vi "GUI_MicrophoneTest.vi"() -> ()   [LabVIEW 2018]
uses:
  C:/Micriphone Test/Microfontest/Peiker_Stepped Sweep Settings.ctl
  <vilib>/addons/_NISVFA/_Shared subVIs/Controls/svc_DSA Channel Settings.ctl
  <vilib>/addons/_NISVFA/_Shared subVIs/Controls/svc_Channel Info.ctl
  <vilib>/addons/_NISVFA/_Shared subVIs/Controls/svc_Engineering Units Text Ring.ctl
  <vilib>/addons/_NISVFA/_Shared subVIs/Controls/svc_Weighting Filter Text Ring.ctl
  <vilib>/addons/Sound and Vibration/svt_Limit Test/SVL Limit Testing (XY) (scalar limits).vi
  <vilib>/addons/Sound and Vibration/svt_Limit Test/SoundVib_LimitTest.lvlib
panel:
  in  "Input Settings.Responce Channel Settings.response channel info":T1={"sensor sensitivity"=1000.0, "engineering units"=1, "dB reference"=1.0, "custom label"="EU", "weighting filter"=0, "pregain"=0.0} {"pregain" format="%.2f"; "weighting filter" items=["Linear", "A-weighting", "B-weighting", "C-weighting", "ITU-R 468-4", "Dolby", "CCITT", "C-message", "Wb", "Wc", "Wd", "We", "Wf", "Wh", "Wj", "Wk", "Wm", "AES17 20 kHz lowpass", "AES17 40 kHz lowpass", "AES17 20 kHz highpass", "AES17 40 kHz highpass"]; "dB reference" format="%^.1e"; "engineering units" items=["custom..."=0, "V"=1, "A"=21, "C"=30, "pC"=31, "s"=32, "-"=29, "Pa"=2, "N"=20, "g"=3, "m/s^2"=4, "m/s"=5, "m"=6, "mm/s"=12, "mm"=13, "micron/s"=14, "micron"=15, "in/s^2"=7, "in/s"=8, "in"=9, "mil/s"=10, "mil"=11, "rad/s^2"=16, "rad/s"=17, "rad"=18, "deg/s^2"=26, "deg/s"=27, "deg"=28, "RPM"=22, "cycle/s^2"=23, "Hz"=24, "cycle"=25, "strain"=19]; "sensor sensitivity" format="%#_5f"}
  out "Fundamental-Response RMS (Engineering unit) 2":T4(graph)={"frequency [Hz]"=[100.0], "amplitude"=[6.209838309826431]} caption="Fundamental-Response RMS"
  out "THD%":cluster{"frequency":dbl[], "THD":dbl[]} {"THD" format="%.2f"; "frequency" format="%.2f"}
  out "THD-Response":cluster{"frequency":dbl[], "THD":dbl[]}(graph)={"frequency"=[100.0], "THD"=[0.18625048733429]} caption="THD"
  out "Fundamental-Response RMS (Engineering unit)":T4
  in  "THD Frequency":dbl
  out "Fundamental-Response RMS (Engineering unit)":T4(graph) caption="harmonics"
  in  "THD Level (dBSpl)":dbl=94.0
  out "Sensitivity(V)":dbl
  in  "Ref.Frequency":dbl=100.0
  out "magnitude first measurement":dbl[](array[numeric])
  in  "Set level (dBSPL)":i32=94
  in  "Peiker_Stepped Sweep Settings":T5={"Input Settings"={"IEPE min time to settle [s]"=5.0, "Responce Channel Settings"={"DSA response channel settings"={"coupling"=10045, "enable IEPE excitation"=FALSE, "IEPE current [mA]"=4.0}, "response channel info"={"sensor sensitivity"=200.0, "engineering units"=2, "dB reference"=2e-05, "custom label"="EU", "weighting filter"=0, "pregain"=0.0}, "AI response settings"={"response channel"="SOUNDACQ/ai1", "max value [V]"=10.0, "min value [V]"=-10.0, "terminal configuration"=-1}}, "Stimulus Channel Settings"={"AI stimulus settings"={"stimulus channel"="SOUNDACQ/ai0", "max value [V]"=0.15, "min value [V]"=-0.15, "terminal configuration"=-1}, "DSA stimulus channel settings"={"coupling"=10045, "enable IEPE excitation"=TRUE, "IEPE current [mA]"=4.0}, "stimulus channel info"={"sensor sensitivity"=11.4, "engineering units"=2, "dB reference"=2e-05, "custom label"="EU", "weighting filter"=0, "pregain"=0.0}}}, "Output Settings"={"AO source settings"={"excitation channel"="SOUNDACQ/ao0", "max value [V]"=10.0, "min value [V]"=-10.0, "terminal configuration"=-1}}} {"Output Settings"."AO source settings"."terminal configuration" items=["Default"=-1, "RSE"=10083, "Differential"=10106, "Pseudodifferential"=12529]; "Output Settings"."AO source settings"."min value [V]" format="%0.2f"; "Output Settings"."AO source settings"."max value [V]" format="%0.2f"; "Input Settings"."Stimulus Channel Settings"."stimulus channel info"."pregain" format="%.2f"; "Input Settings"."Stimulus Channel Settings"."stimulus channel info"."weighting filter" items=["Linear", "A-weighting", "B-weighting", "C-weighting", "ITU-R 468-4", "Dolby", "CCITT", "C-message", "Wb", "Wc", "Wd", "We", "Wf", "Wh", "Wj", "Wk", "Wm", "AES17 20 kHz lowpass", "AES17 40 kHz lowpass", "AES17 20 kHz highpass", "AES17 40 kHz highpass"]; "Input Settings"."Stimulus Channel Settings"."stimulus channel info"."dB reference" format="%^.1e"; "Input Settings"."Stimulus Channel Settings"."stimulus channel info"."engineering units" items=["custom..."=0, "V"=1, "A"=21, "C"=30, "pC"=31, "s"=32, "-"=29, "Pa"=2, "N"=20, "g"=3, "m/s^2"=4, "m/s"=5, "m"=6, "mm/s"=12, "mm"=13, "micron/s"=14, "micron"=15, "in/s^2"=7, "in/s"=8, "in"=9, "mil/s"=10, "mil"=11, "rad/s^2"=16, "rad/s"=17, "rad"=18, "deg/s^2"=26, "deg/s"=27, "deg"=28, "RPM"=22, "cycle/s^2"=23, "Hz"=24, "cycle"=25, "strain"=19]; "Input Settings"."Stimulus Channel Settings"."stimulus channel info"."sensor sensitivity" format="%#_5f"; "Input Settings"."Stimulus Channel Settings"."DSA stimulus channel settings"."IEPE current [mA]" format="%.1f"; "Input Settings"."Stimulus Channel Settings"."DSA stimulus channel settings"."coupling" items=["AC"=10045, "DC"=10050, "GND"=10066]; "Input Settings"."Stimulus Channel Settings"."AI stimulus settings"."terminal configuration" items=["Default"=-1, "RSE"=10083, "NRSE"=10078, "Differential"=10106, "Pseudodifferential"=12529]; "Input Settings"."Stimulus Channel Settings"."AI stimulus settings"."min value [V]" format="%.2f"; "Input Settings"."Stimulus Channel Settings"."AI stimulus settings"."max value [V]" format="%.2f"; "Input Settings"."Responce Channel Settings"."AI response settings"."terminal configuration" items=["Default"=-1, "RSE"=10083, "NRSE"=10078, "Differential"=10106, "Pseudodifferential"=12529]; "Input Settings"."Responce Channel Settings"."AI response settings"."min value [V]" format="%.2f"; "Input Settings"."Responce Channel Settings"."AI response settings"."max value [V]" format="%.2f"; "Input Settings"."Responce Channel Settings"."response channel info"."pregain" format="%.2f"; "Input Settings"."Responce Channel Settings"."response channel info"."weighting filter" items=["Linear", "A-weighting", "B-weighting", "C-weighting", "ITU-R 468-4", "Dolby", "CCITT", "C-message", "Wb", "Wc", "Wd", "We", "Wf", "Wh", "Wj", "Wk", "Wm", "AES17 20 kHz lowpass", "AES17 40 kHz lowpass", "AES17 20 kHz highpass", "AES17 40 kHz highpass"]; "Input Settings"."Responce Channel Settings"."response channel info"."dB reference" format="%^.1e"; "Input Settings"."Responce Channel Settings"."response channel info"."engineering units" items=["custom..."=0, "V"=1, "A"=21, "C"=30, "pC"=31, "s"=32, "-"=29, "Pa"=2, "N"=20, "g"=3, "m/s^2"=4, "m/s"=5, "m"=6, "mm/s"=12, "mm"=13, "micron/s"=14, "micron"=15, "in/s^2"=7, "in/s"=8, "in"=9, "mil/s"=10, "mil"=11, "rad/s^2"=16, "rad/s"=17, "rad"=18, "deg/s^2"=26, "deg/s"=27, "deg"=28, "RPM"=22, "cycle/s^2"=23, "Hz"=24, "cycle"=25, "strain"=19]; "Input Settings"."Responce Channel Settings"."response channel info"."sensor sensitivity" format="%#_5f"; "Input Settings"."Responce Channel Settings"."DSA response channel settings"."IEPE current [mA]" format="%.1f"; "Input Settings"."Responce Channel Settings"."DSA response channel settings"."coupling" items=["AC"=10045, "DC"=10050, "GND"=10066]; "Input Settings"."IEPE min time to settle [s]" format="%.1f"}
  in  "integration time":T7={"integration time [s]"=0.015599999576807022, "integration cycles"=5} {"integration cycles" min=2; "integration time [s]" format="%.2p"}
  in  "settling time":T8={"settle time [s]"=0.015599999576807022, "settle cycles"=5} {"settle time [s]" format="%.2p"}
  in  "Frequency List":T9(array[cluster])
  in  "Amplitude [V]":dbl=0.2
  # "Achtung immer DUT Microphone einstellen"
  # "Generate frequency table"
  # "Versuchsweise eine FFT durchgeführt"
  # "Microfon"
  # "Signal direkt später DUT AI1"
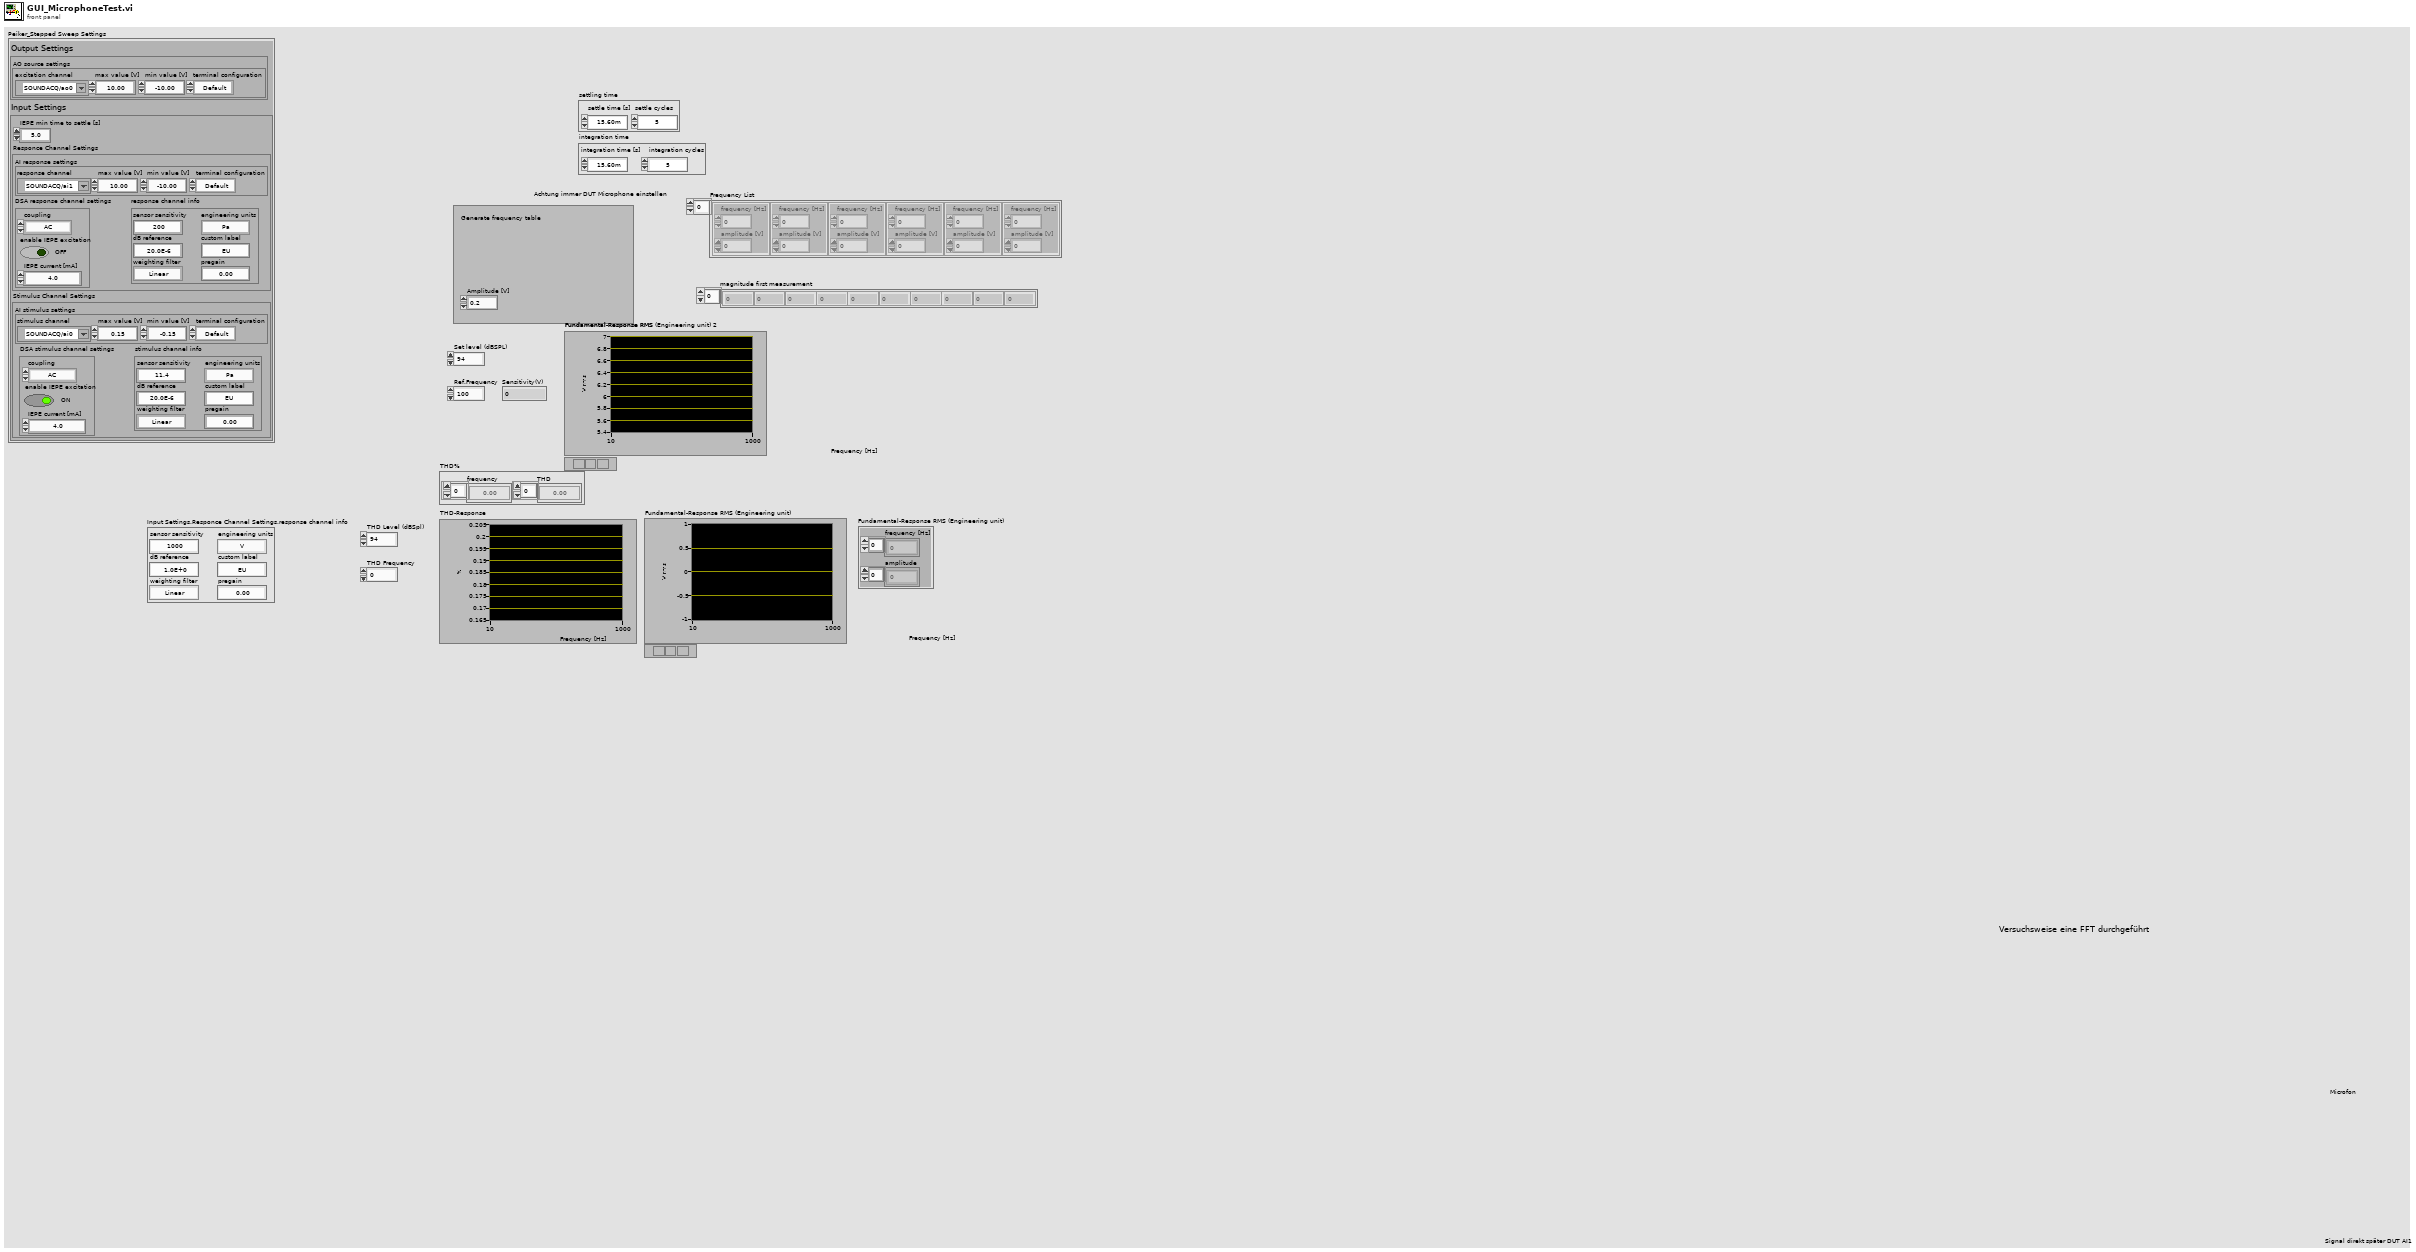
[diagram p1: front panel]
types:
  T1 = typedef "svc_Channel Info.ctl" = cluster{"sensor sensitivity":dbl, "engineering units":T2, "dB reference":dbl, "custom label":string, "weighting filter":T3, "pregain":dbl}
  T2 = typedef "svc_Engineering Units Text Ring.ctl" = u16
  T3 = typedef "svc_Weighting Filter Text Ring.ctl" = u16
  T4 = cluster{"frequency [Hz]":dbl[], "amplitude":dbl[]}
  T5 = typedef "Peiker_Stepped Sweep Settings.ctl" = cluster{"Input Settings":cluster{"IEPE min time to settle [s]":dbl, "Responce Channel Settings":cluster{"DSA response channel settings":T6, "response channel info":T1, "AI response settings":cluster{"response channel":tag, "max value [V]":dbl, "min value [V]":dbl, "terminal configuration":i32}}, "Stimulus Channel Settings":cluster{"AI stimulus settings":cluster{"stimulus channel":tag, "max value [V]":dbl, "min value [V]":dbl, "terminal configuration":i32}, "DSA stimulus channel settings":T6, "stimulus channel info":T1}}, "Output Settings":cluster{"AO source settings":cluster{"excitation channel":tag, "max value [V]":dbl, "min value [V]":dbl, "terminal configuration":i32}}}
  T6 = typedef "svc_DSA Channel Settings.ctl" = cluster{"coupling":i32, "enable IEPE excitation":bool, "IEPE current [mA]":dbl}
  T7 = cluster{"integration time [s]":dbl, "integration cycles":i32}
  T8 = cluster{"settle time [s]":dbl, "settle cycles":i32}
  T9 = cluster{"frequency [Hz]":dbl, "amplitude [V]":dbl}[]
  T10 = cluster{"frequency [Hz]":dbl, "amplitude [V]":dbl}
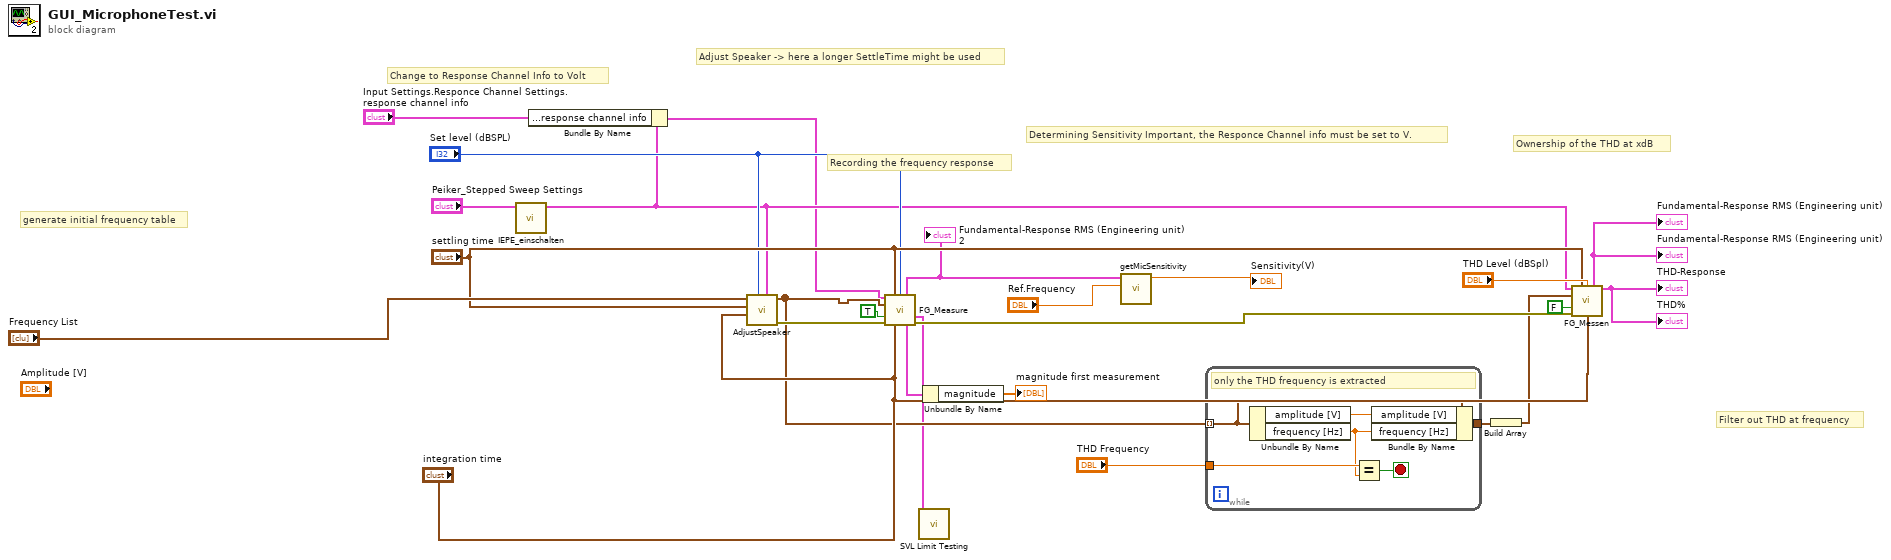
[diagram p0: block diagram]
diagram:
  # "Change to Response Channel Info to Volt"
  # "Adjust Speaker -> here a longer SettleTime might be used"
  # "Filter out THD at frequency"
  # "Ownership of the THD at xdB"
  # "Determining Sensitivity Important, the Responce Channel info must be set to V."
  # "Recording the frequency response"
  # "generate initial frequency table"
  n1 = call "IEPE_einschalten.vi"("Peiker_Stepped Sweep Settings"="Peiker_Stepped Sweep Settings") -> ("Peiker_Stepped Sweep Settings (IEPE Settle-Time=0)"=w2:T5)  [unwired: 9 in, 1 out]
  n2 = Bundle By Name(cluster=w2, "Input Settings.Responce Channel Settings.response channel info"="Input Settings.Responce Channel Settings.response channel info") -> (w1:T5)
  n3 = call "AdjustSpeaker.vi"("Peiker_Stepped Sweep Settings"=w2, "Set Level(dBSPL)"="Set level (dBSPL)", "integration time"="integration time", "settling time"="settling time", "Frequency List"="Frequency List") -> ("error out"=w11:errorcluster, "Corrected frequency list"=w10:T9)  [unwired: 4 in, 1 out]
  n4 = call "FG_Measure.vi"("Peiker_Stepped Sweep Settings"=w1, "settling time"="settling time", "FrequencyList Output Level (dBSPL)"="Set level (dBSPL)", "frequency list Input"=w10, "true = measure several times"=TRUE ("true=mehrfach Messen"), "error in (no error)"=w11, "integration time"="integration time") -> ("Fundamental-Response"=w4:T4, "Response Level"=w5:cluster{"frequency":dbl[], "magnitude":dbl[]}, "Stimulus Level"=w23:cluster{"frequency":dbl[], "magnitude":dbl[]}, "error out"=w15:errorcluster)  [unwired: 3 in, 2 out]
  "Fundamental-Response RMS (Engineering unit) 2" <- w4
  n5 = call-poly <vilib>:"SVL Limit Testing.vi"("signal in"=w5) -> ()  [unwired: 7 in, 4 out]
  n6 = Unbundle By Name(w23) -> ("magnitude"=→"magnitude first measurement":dbl[])
  n7 = call "getMicSensitivity.vi"("Ref.Frequenz"="Ref.Frequency", "fundamental amplitude"=w4) -> ("Sensitivity/V"=→"Sensitivity(V)":dbl)  [unwired: 9 in]
  n8 = while {
    tunnel: w10 -> [w29] mode=indexing
    tunnel: "THD Frequency" -> [w30]
    tunnel: [w26] -> w8
    stop <- w31 stop-if-true
    # "only the THD frequency is extracted"
    n9 = Unbundle By Name(w29) -> ("amplitude [V]"=w27:dbl, "frequency [Hz]"=w28:dbl)
    n10 = Equal?(x=w30, y=w28) -> (x = y?=w31:bool)
    n11 = Bundle By Name(cluster=w29, "amplitude [V]"=w27, "frequency [Hz]"=w28) -> (w26:T10)
  }
  n12 = Build Array(w8) -> (w7:T9)
  n13 = call "FG_Messen.vi"("Peiker_Stepped Sweep Settings"=w2, "settling time"="settling time", "FrequencyList Output Level (dBSPL)"="THD Level (dBSpl)", "frequency list Input"=w7, "true=mehrfach Messen"=FALSE, "error in (no error)"=w15, "integration time"="integration time") -> ("Fundamental-Response"=→"Fundamental-Response RMS (Engineering unit)" →"Fundamental-Response RMS (Engineering unit)":T4, "THD-Response"=→"THD-Response" →"THD%":cluster{"frequency":dbl[], "THD":dbl[]})  [unwired: 3 in, 4 out]
